vi "ESP32 Continuous Serial Write and Read - Modified.vi"() -> ()   [LabVIEW 2022 SP3]
doc: "This example performs writes and reads on a serial port, as directed by the user. You can press the Write and Read buttons, and change the Read Count, while the example is running.\n\nThe parameters set for the serial port must match the parameters of the connected instrument or device. In this example, the Read Count parameter specifies the number of bytes that the serial port reads. If there were more bytes at the port than the specified number, those bytes would not be read. If there were less bytes at the port than the specified number, you would receive a timeout error.\n\nThis example expands upon the flow control options for XON and XOFF, allowing the user to choose those control characters. Also, the user can enable or disable a termination character. Some devices require a termination character in order to identify the end of command strings. Some devices send a termination character to signify the end of data to be read. This example shows how you can end the Read operation once a termination character is detected in the buffer and/or append a termination character at the end of the Write data."
uses:
  Serial - Settings.ctl
  Serial - XON-XOFF Characters.ctl
  Serial - ASCII Characters.ctl
  ESP32-PSOC-State Machine.ctl
  <vilib>/Instr/_visa.llb/VISA Flush IO Buffer Mask.ctl
  <vilib>/Instr/_visa.llb/VISA Configure Serial Port (Instr).vi
panel:
  in  "Difficulty":T1
  out "error":bool
  out "Connected":bool
  out "Serial Settings:Number of Bytes at Serial Port":u32
  out "Response 2":string
  in  "Toggle LED":bool
  in  "Enum":T2
  in  "Termination Character":u8=10 format="%.0x"
  in  "End Write on Termination Character?":bool=TRUE
  in  "Stop":bool
  out "Read Count":u32=1000
  out "Response":string
  in  "XON/XOFF Characters":T3={"XON"=enum."DC1", "XOFF"=enum."DC3"}
  in  "Serial Settings":T5={"baud rate"=115200, "data bits"=8, "parity"=enum."None", "stop bits"=10, "flow control"=0} {"flow control" items=["None"=0, "XON/XOFF"=1, "RTS/CTS"=2, "DTR/DSR"=4]; "stop bits" items=["1.0"=10, "1.5"=15, "2.0"=20]; "data bits" min=5 max=8 step=1; "baud rate" items=["75"=75, "110"=110, "134"=134, "150"=150, "300"=300, "600"=600, "1200"=1200, "1800"=1800, "2400"=2400, "4800"=4800, "7200"=7200, "9600"=9600, "14400"=14400, "19200"=19200, "28800"=28800, "38400"=38400, "56000"=56000, "57600"=57600, "115200"=115200, "128000"=128000, "230400"=230400]}
  in  "End Read on Termination Character?":bool=TRUE
  in  "VISA resource name":refnum<visa-resource-name>="COM4"
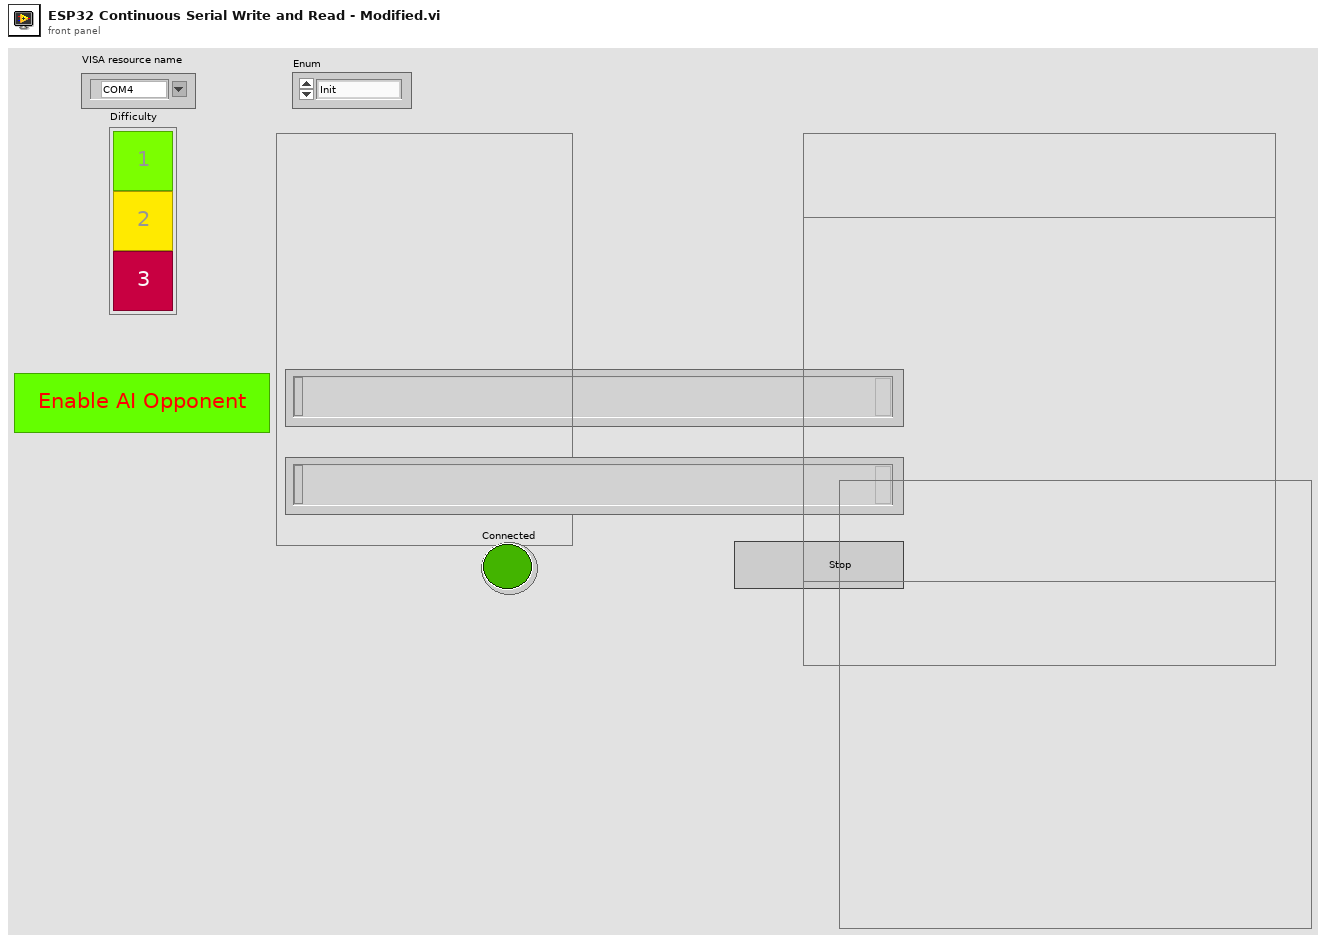
[diagram p1: front panel]
types:
  T1 = cluster{"Command A":bool, "Command B":bool, "Command C":bool}
  T2 = typedef "ESP32-PSOC-State Machine.ctl" = enum8{"Init", "Connect", "idle", "send", "wait", "receive", "que", "error", "exit"}
  T3 = typedef "Serial - XON-XOFF Characters.ctl" = cluster{"XON":T4, "XOFF":T4}
  T4 = typedef "Serial - ASCII Characters.ctl" = enum16{"NUL", "SOH", "STX", "ETX", "EOT", "ENQ", "ACK", "BEL", "BS", "HT", "LF", "VT", "FF", "CR", "SO", "SI", "DLE", "DC1", "DC2", "DC3", "DC4", "NAK", "SYN", "ETB", "CAN", "EM", "SUB", "ESC", "FS", "GS", "RS", "US", "SP", "!", "\"", "#", "$", "%", "&", "'", "(", ")", "*", "+", ",", "- (-)", ".", "/", "0", "1", "2", "3", "4", "5", "6", "7", "8", "9", ":", ";", "<", "=", ">", "?", "@", "A", "B", "C", "D", "E", "F", "G", "H", "I", "J", "K", "L", "M", "N", "O", "P", "Q", "R", "S", "T", "U", "V", "W", "X", "Y", "Z", "[", "\\", "]", "^", "_", "`", "a", "b", "c", "d", "e", "f", "g", "h", "i", "j", "k", "l", "m", "n", "o", "p", "q", "r", "s", "t", "u", "v", "w", "x", "y", "z", "{", "|", "}", "~"}
  T5 = typedef "Serial - Settings.ctl" = cluster{"baud rate":u32, "data bits":u16, "parity":enum16{"None", "Odd", "Even", "Mark", "Space"}, "stop bits":u16, "flow control":u16}
  T6 = typedef "VISA Flush IO Buffer Mask.ctl" = u16
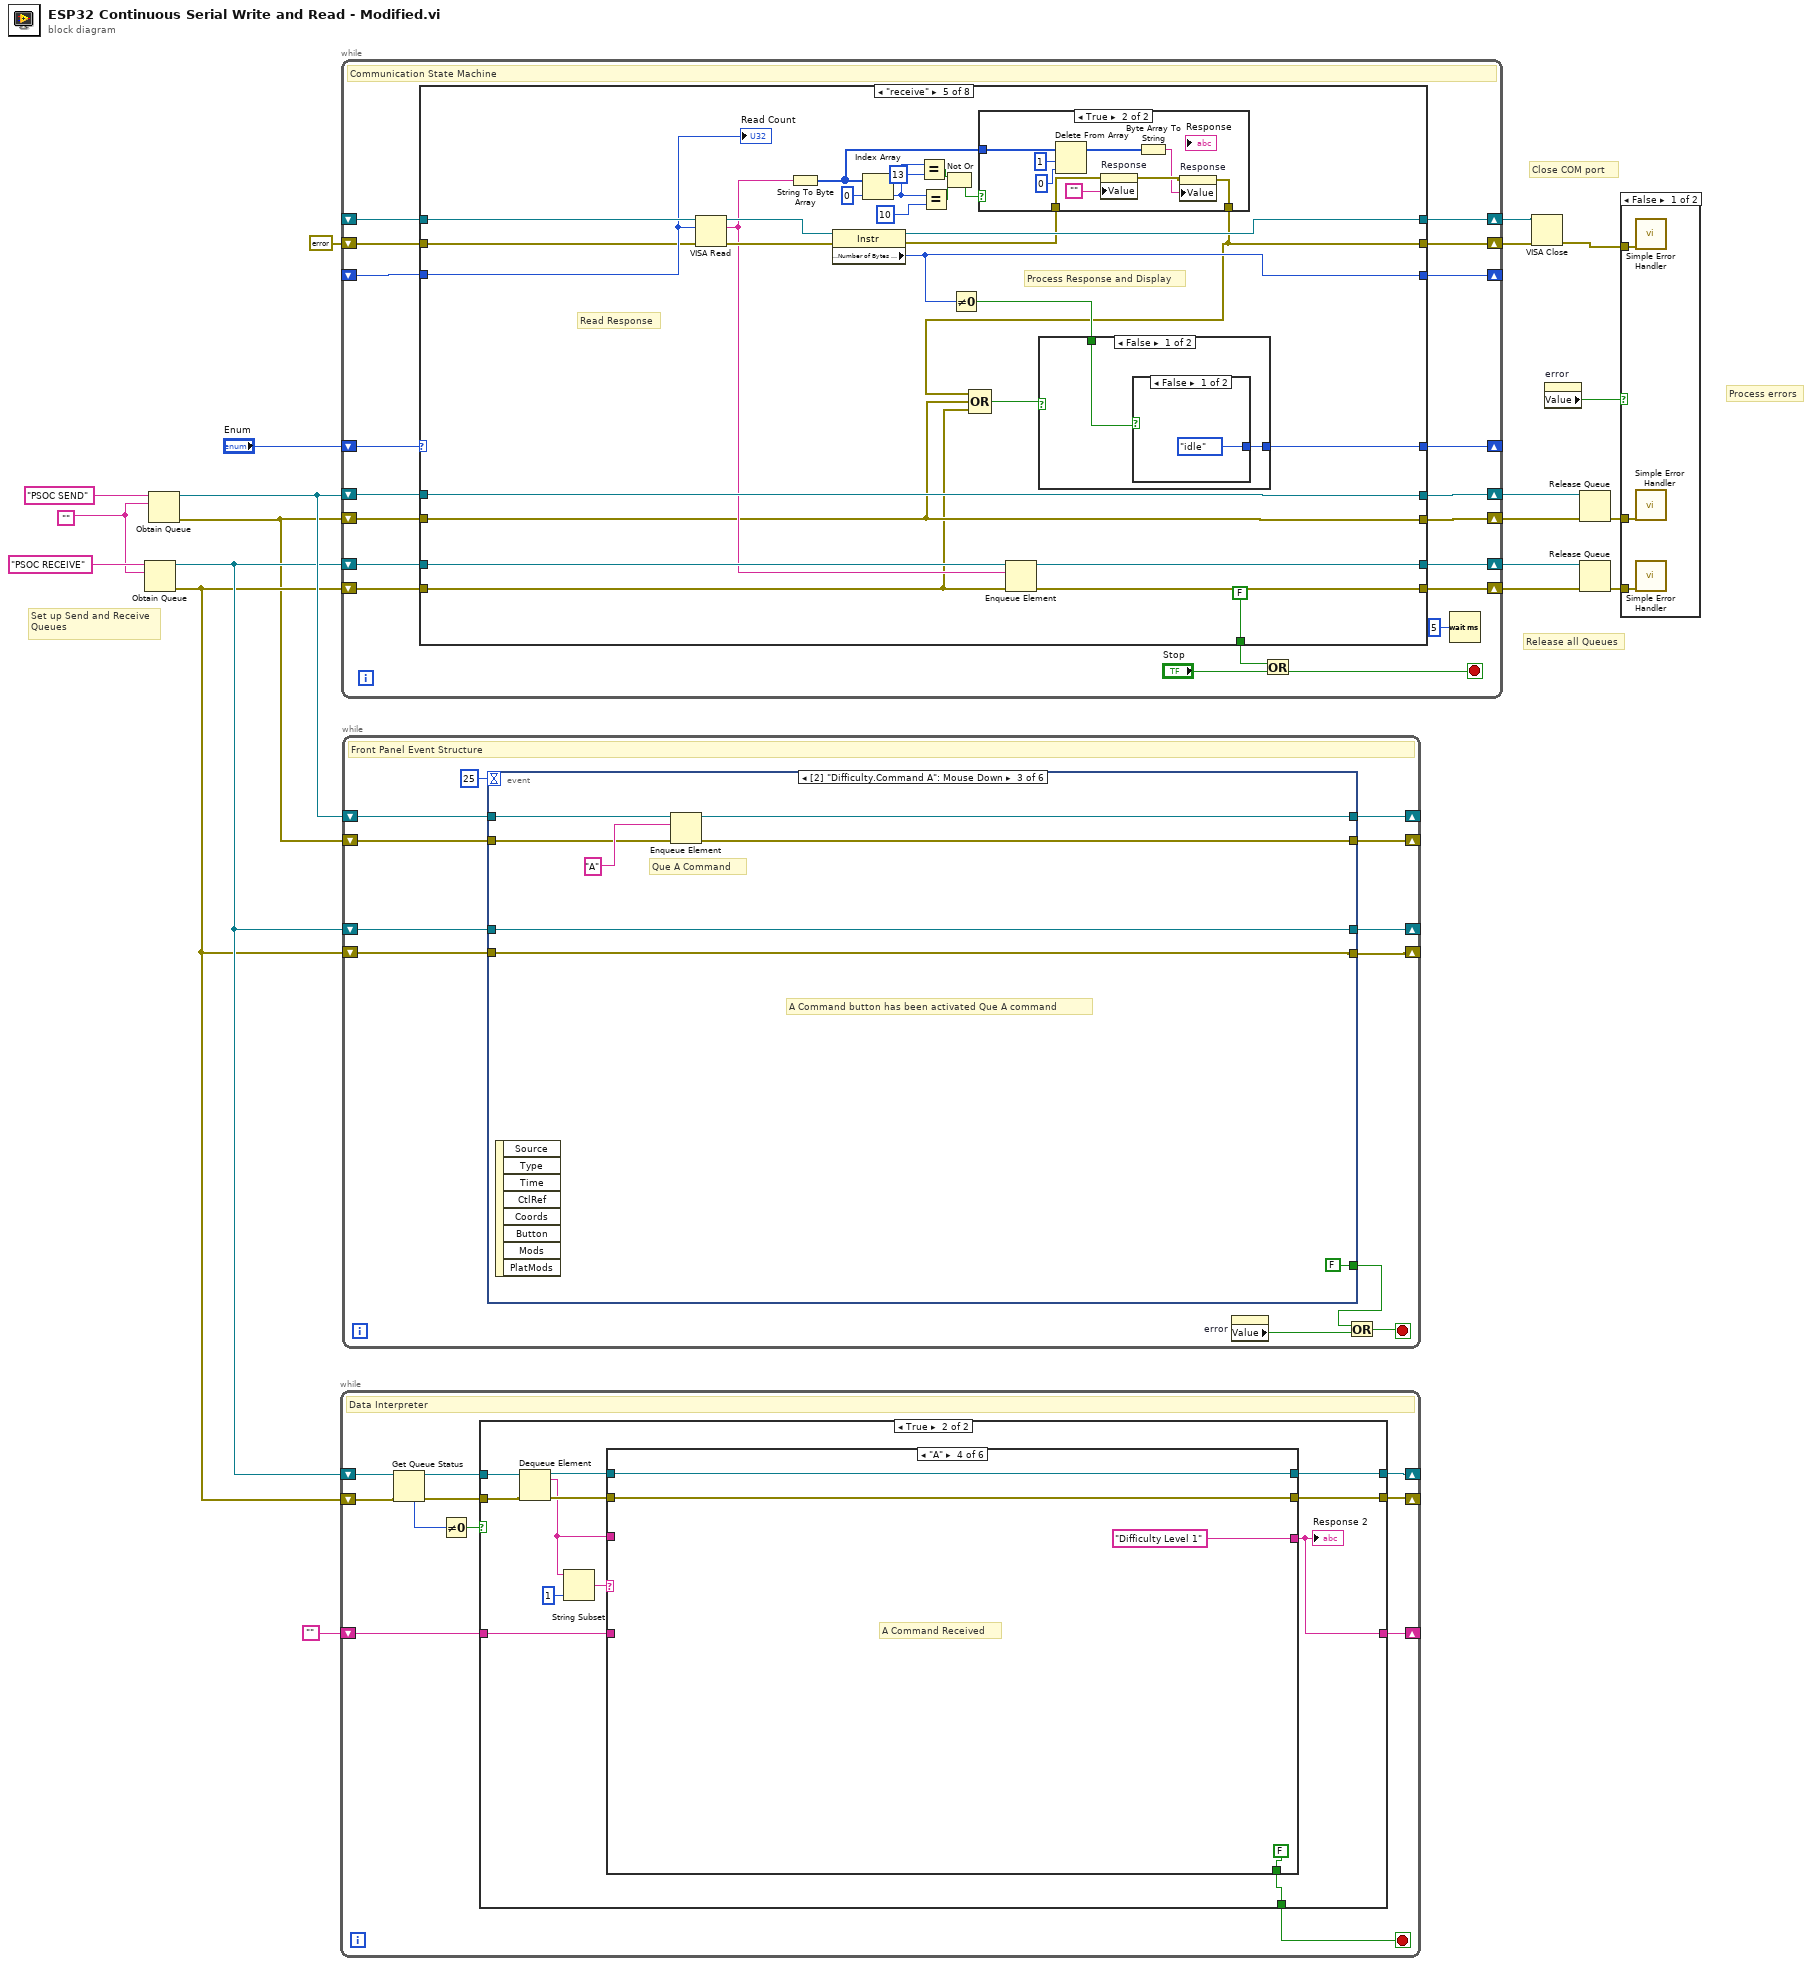
[diagram p0: block diagram]
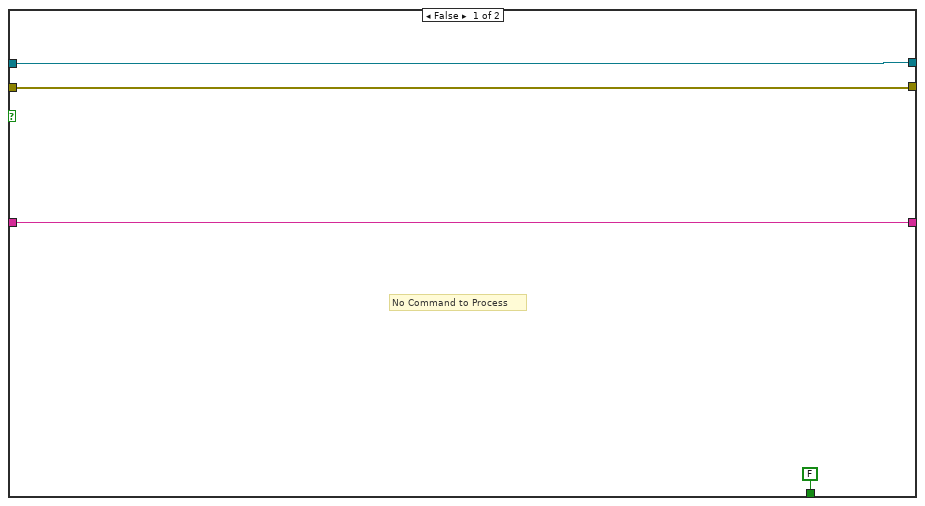
[diagram p3: hidden frame]
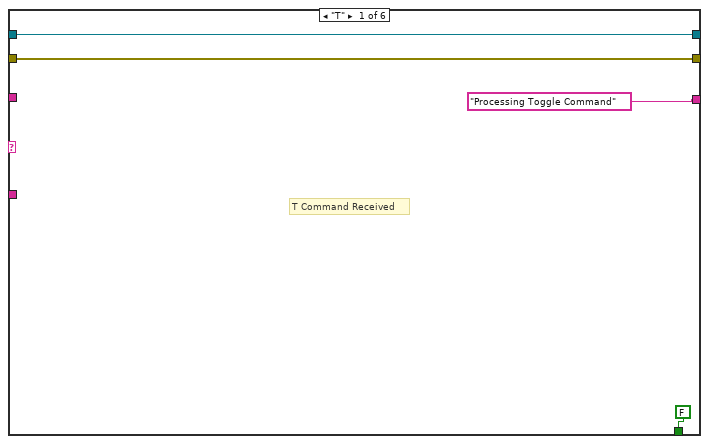
[diagram p4: hidden frame]
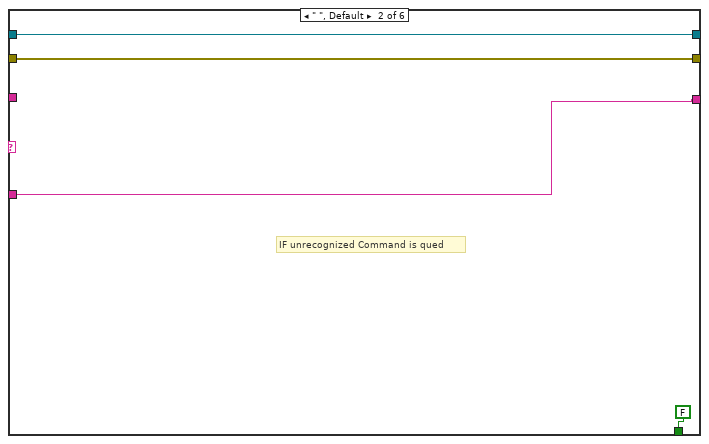
[diagram p5: hidden frame]
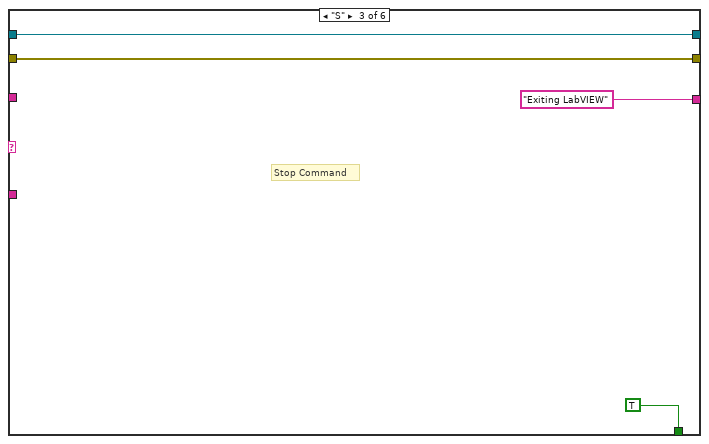
[diagram p6: hidden frame]
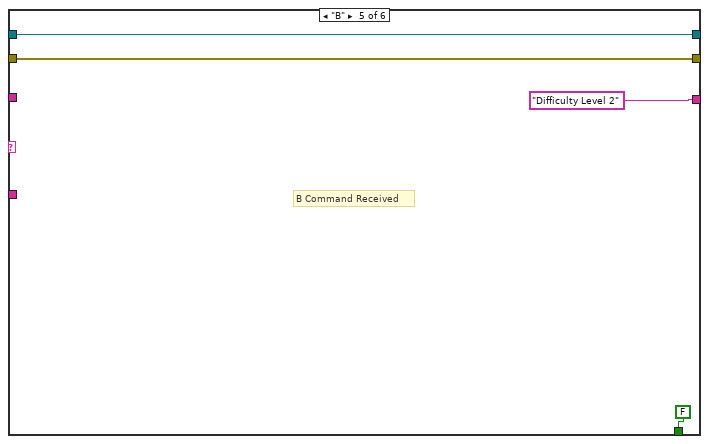
[diagram p7: hidden frame]
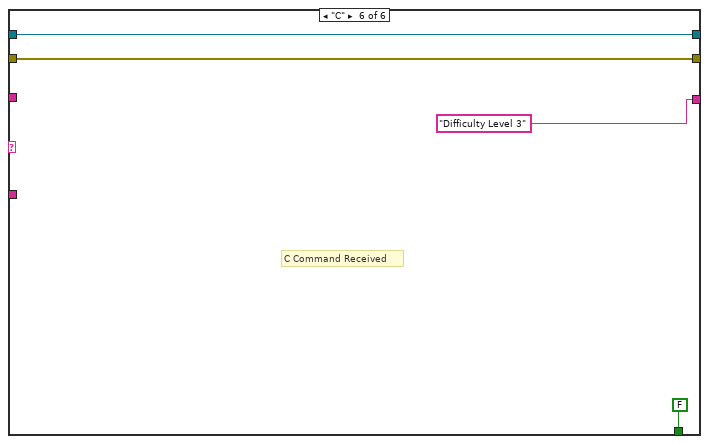
[diagram p8: hidden frame]
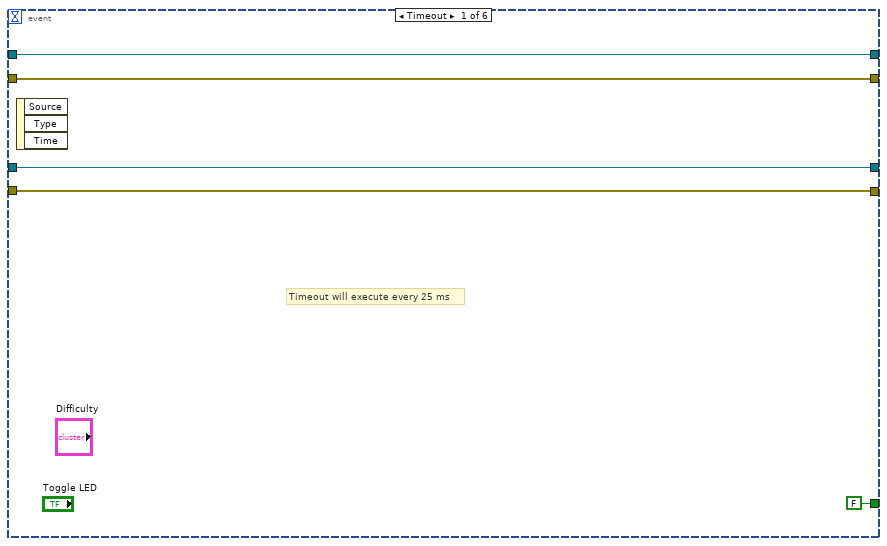
[diagram p9: hidden frame]
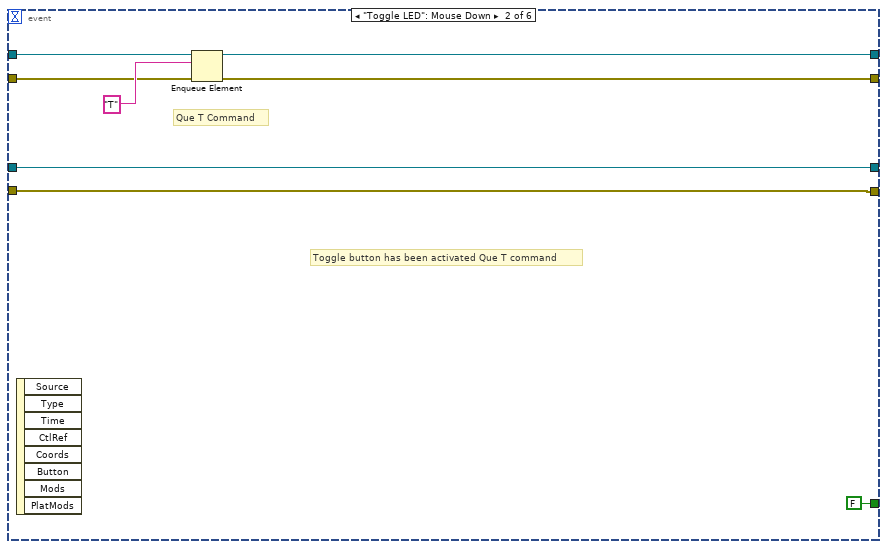
[diagram p10: hidden frame]
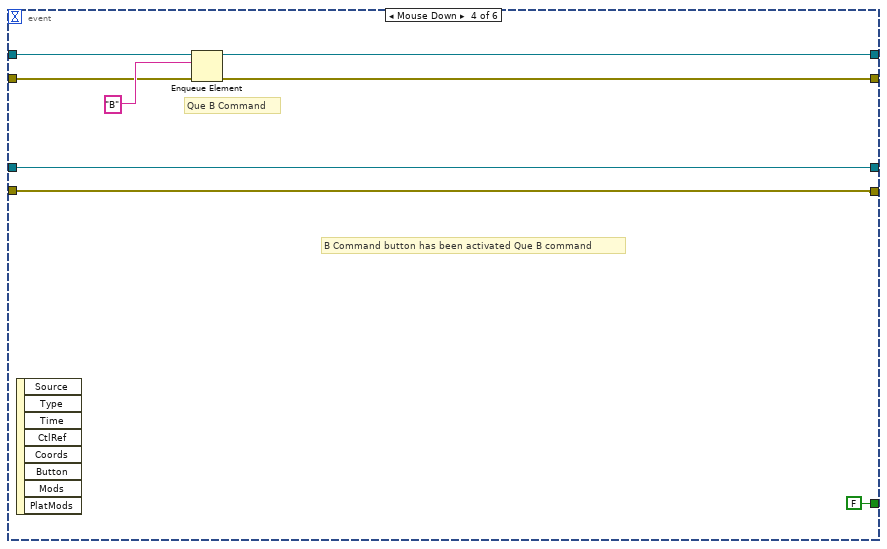
[diagram p11: hidden frame]
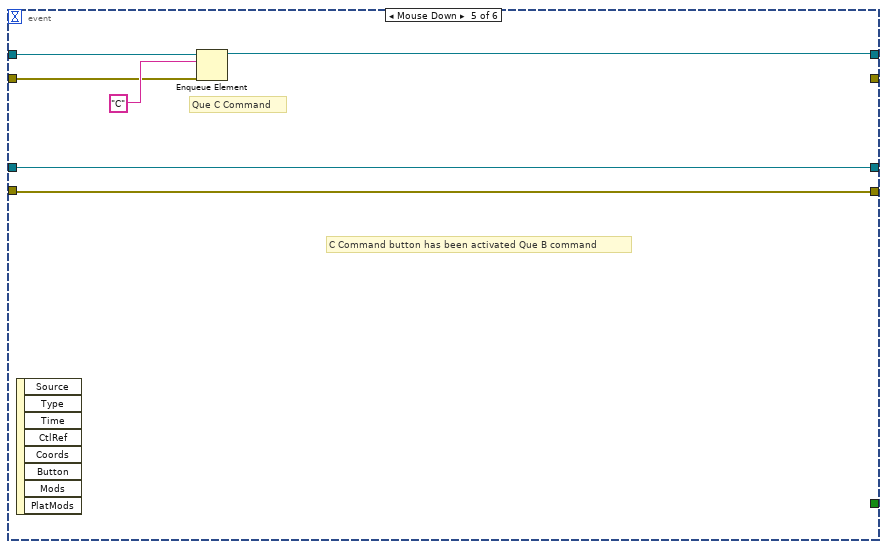
[diagram p12: hidden frame]
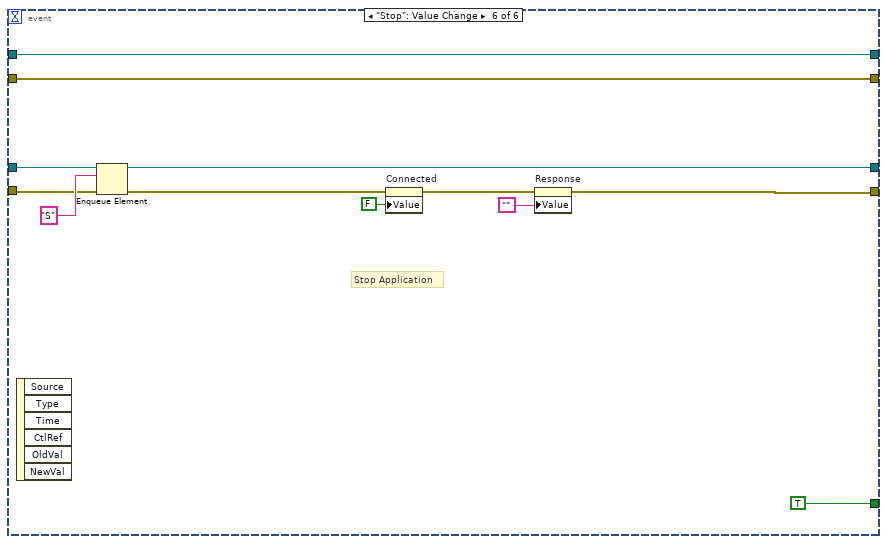
[diagram p13: hidden frame]
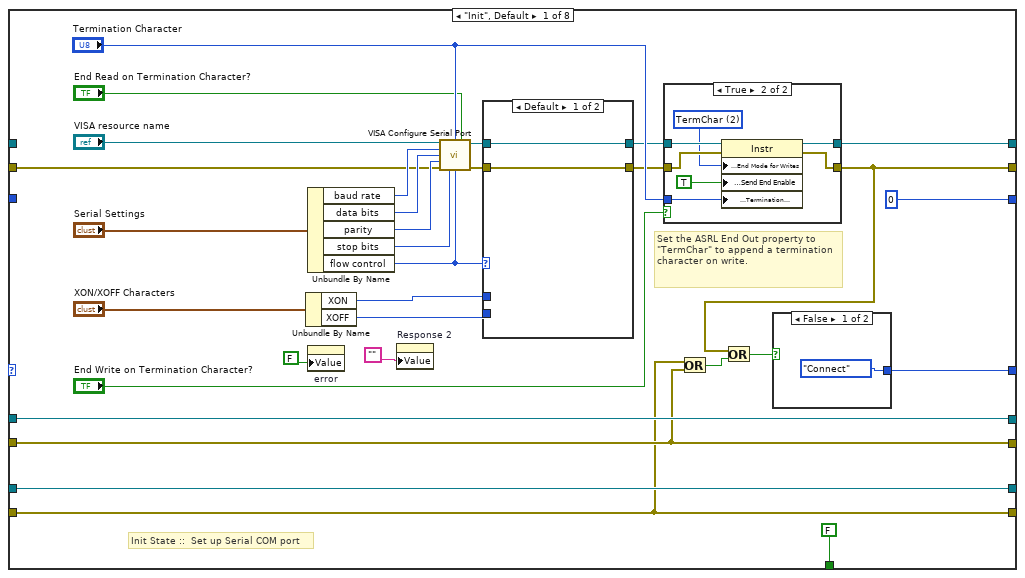
[diagram p14: hidden frame]
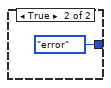
[diagram p15: hidden frame]
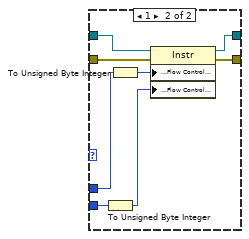
[diagram p17: hidden frame]
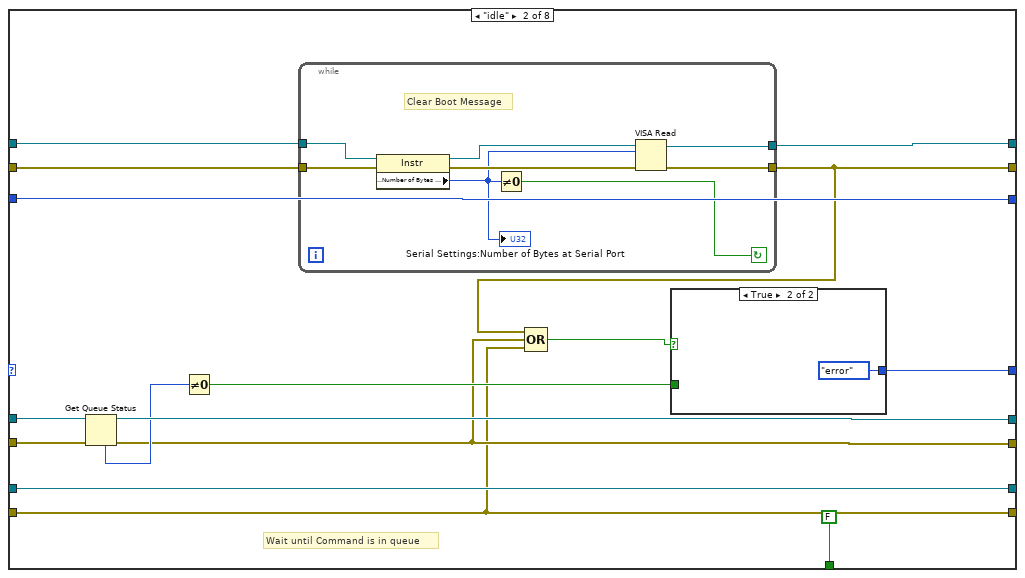
[diagram p18: hidden frame]
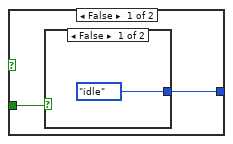
[diagram p19: hidden frame]
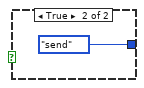
[diagram p20: hidden frame]
diagram:
  w10 = ""
  # "Process errors"
  # "Release all Queues"
  # "Close COM port"
  # "Set up Send and Receive\nQueues"
  n1 = Obtain Queue(name (unnamed)="PSOC RECEIVE", element data type=w10) -> (queue out=w9:refnum<queue>, error out=w8:errorcluster)  [unwired: 3 in, 1 out]
  n2 = Obtain Queue(name (unnamed)="PSOC SEND", element data type=w10) -> (queue out=w12:refnum<queue>, error out=w2:errorcluster)  [unwired: 3 in, 1 out]
  n3 = while {
    shift-right: [w25] -> _
    shift-left: w9 -> [w31]
    shift-right: [w24] -> _
    shift-left: w8 -> [w30]
    shift-right: [w22] -> _
    shift-left: "" -> [w21]
    stop <- w23 stop-if-true
    # "Data Interpreter"
    n4 = Get Queue Status(queue=w31, error in (no error)=w30) -> (queue out=w27:refnum<queue>, error out=w26:errorcluster, # elements in queue=w29:i32)  [unwired: 1 in, 5 out]
    n5 = Not Equal To 0?(x=w29) -> (x != 0?=w28:bool)
    n6 = case shown="True" w28 {
      tunnel: w27 -> [w35 w47]
      tunnel: w26 -> [w34 w46]
      tunnel: [w35 w41] -> w25
      tunnel: [w34 w40] -> w24
      tunnel: [FALSE w39] -> w23
      tunnel: [w32 w37] -> w22
      tunnel: w21 -> [w32 w36]
      frame False {
        # "No Command to Process"
      }
      frame True {
        n7 = Dequeue Element(queue=w47, error in (no error)=w46) -> (queue out=w45:refnum<queue>, element=w38:string, error out=w44:errorcluster)  [unwired: 1 in, 1 out]
        n8 = String Subset(string=w38, length (rest)=1 ("length (rest)")) -> (substring=w42:string)  [unwired: 1 in]
        n9 = case shown="\"A\"" w42 {
          tunnel: w45 -> [w51 w55 w59 w63 w67 w69]
          tunnel: w44 -> [w50 w54 w58 w62 w66 w70]
          tunnel: [w51 w55 w59 w63 w67 w69] -> w41
          tunnel: [w50 w54 w58 w62 w66 w70] -> w40
          tunnel: w38 -> [_ _ _ _ _ _]
          tunnel: [FALSE FALSE TRUE FALSE FALSE FALSE] -> w39
          tunnel: ["Processing Toggle Command" w52 "Exiting LabVIEW" "Difficulty Level 1" "Difficulty Level 2" "Difficulty Level 3"] -> w37
          tunnel: w36 -> [_ w52 _ _ _ _]
          frame "T" {
            # "T Command Received"
          }
          frame " ", Default {
            # "IF unrecognized Command is qued"
          }
          frame "S" {
            # "Stop Command"
          }
          frame "A" {
            # "A Command Received"
          }
          frame "B" {
            # "B Command Received"
          }
          frame "C" {
            # "C Command Received"
          }
        }
        "Response 2" <- w37
      }
    }
  }
  n10 = while {
    shift-right: [w83] -> w20
    shift-left: w12 -> [w91]
    shift-right: [w82] -> w18
    shift-left: w2 -> [w90]
    shift-right: [w81] -> w19
    shift-left: w9 -> [w89]
    shift-right: [w80] -> w15
    shift-left: w8 -> [w88]
    shift-right: [w75] -> _
    shift-left: "Enum" -> [w74]
    shift-right: [w87] -> w14
    shift-left: _ -> [w84]
    shift-right: [w86] -> w13
    shift-left: errorcluster {"status"=FALSE, "code"=0, "source"=""} ("error out") -> [w85]
    shift-right: [w79] -> _
    shift-left: _ -> [w78]
    stop <- w73 stop-if-true
    # "Communication State Machine"
    n11 = case shown="\"receive\"" w74 {
      selector: w74 -> [_ _ _ _ _ _ w291 _]
      tunnel: [w121 w157 w196 w213 w250 w275 w290 w313] -> w83
      tunnel: [w95 w147 w187 w207 w232 w272 w289 w312] -> w82
      tunnel: [w101 w155 w188 w216 w251 ESP32-PSOC-State_Machine."exit" ("Enum") w291 ESP32-PSOC-State_Machine."idle" ("Enum")] -> w75
      tunnel: w91 -> [w121 w159 w198 w213 w250 w275 w290 w313]
      tunnel: w90 -> [w95 w158 w197 w207 w232 w272 w289 w312]
      tunnel: w89 -> [w122 w153 w195 w210 w245 w274 w288 w311]
      tunnel: w88 -> [w94 w146 w186 w206 w231 w271 w279 w310]
      tunnel: [w103 w150 w182 w215 w240 w277 w294 w315] -> w87
      tunnel: [w97 w148 w183 w208 w233 w273 w293 w316] -> w86
      tunnel: w85 -> [w99 w149 w191 w214 w235 w273 w293 w317]
      tunnel: w84 -> [_ w151 w193 w204 w248 w277 w294 w318]
      tunnel: [w122 w153 w195 w210 w243 w274 w286 w311] -> w81
      tunnel: [w94 w146 w186 w206 w244 w271 w282 w310] -> w80
      tunnel: [u32 0 ("Bytes at Port") w152 w194 w212 w246 w276 w292 w314] -> w79
      tunnel: w78 -> [_ w152 w194 _ w242 w276 w292 w314]
      tunnel: [FALSE FALSE FALSE FALSE FALSE FALSE TRUE FALSE] -> w72
      frame "Init", Default {
        # "Init State ::  Set up Serial COM port"
        # "Set the ASRL End Out property to \"TermChar\" to append a termination character on write."
        n12 = Unbundle By Name("XON/XOFF Characters") -> ("XON"=w115:T4, "XOFF"=w116:T4)
        n13 = Unbundle By Name("Serial Settings") -> ("baud rate"=w111:u32, "data bits"=w110:u16, "parity"=w109:enum16{"None", "Odd", "Even", "Mark", "Space"}, "stop bits"=w108:u16, "flow control"=w114:u16)
        n14 = property on="error" class="Bool (strict)"("Value"=FALSE ("error")) -> ()  [unwired: 2 in, 2 out]
        n15 = property on="Response 2" class="Str"("Value"="") -> ()  [unwired: 2 in, 2 out]
        n16 = call-poly "VISA Configure Serial Port"("VISA resource name"="VISA resource name", "termination char\n(0xA = '\\n' = LF)"="Termination Character", "Enable Termination\nChar (T)"="End Read on Termination Character?", "baud rate (9600)"=w111, "data bits (8)"=w110, "parity (0:none)"=w109, "error in (no error)"=w99, "stop bits (10: 1 bit)"=w108, "flow control (0:none)"=w114) -> ("VISA resource name out"=w107:refnum<visa-resource-name>, "error out"=w106:errorcluster)  [unwired: 1 in, 4 out]
        n17 = case shown="Default" w114 {
          tunnel: [w134 w143] -> w117
          tunnel: [w135 w142] -> w118
          tunnel: w106 -> [w134 w141]
          tunnel: w107 -> [w135 w140]
          tunnel: w115 -> [_ w139]
          tunnel: w116 -> [_ w138]
          frame Default {
          }
          frame 1 {
            n18 = To Unsigned Byte Integer(number=w138) -> (unsigned 8bit integer=w137:u8)
            n19 = To Unsigned Byte Integer(number=w139) -> (unsigned 8bit integer=w136:u8)
            n20 = property class="Instr"(reference=w140, error in=w141, "Serial Settings:Flow Control XON Character"=w136, "Serial Settings:Flow Control XOFF Character"=w137) -> (reference out=w142:refnum<visa-resource-name>, error out=w143:errorcluster)
          }
        }
        n21 = case shown="True" "End Write on Termination Character?" {
          tunnel: w118 -> [w125 w133]
          tunnel: w117 -> [w126 w132]
          tunnel: [w125 w131] -> w103
          tunnel: [w126 w130] -> w97
          tunnel: "Termination Character" -> [_ w128]
          frame False {
          }
          frame True {
            w129 = u16 2 items=["None", "LastBit", "TermChar", "Break"] ("Serial Settings:Serial End Mode for Writes")
            n22 = property class="Instr"(reference=w133, error in=w132, "Serial Settings:End Mode for Writes"=w129, "Message Based Settings:Send End Enable"=TRUE, "Message Based Settings:Termination Character"=w128) -> (reference out=w131:refnum<visa-resource-name>, error out=w130:errorcluster)
          }
        }
        n23 = Or(x=w94, y=w95) -> (x .or. y?=w96:bool)
        n24 = Or(x=w97, y=w96) -> (x .or. y?=w98:bool)
        n25 = case shown="False" w98 {
          tunnel: [ESP32-PSOC-State_Machine."Connect" ("Enum") ESP32-PSOC-State_Machine."error" ("Enum")] -> w101
          frame False {
          }
          frame True {
          }
        }
      }
      frame "idle" {
        # "Wait until Command is in queue"
        n26 = Get Queue Status(queue=w159, error in (no error)=w158) -> (queue out=w157:refnum<queue>, error out=w147:errorcluster, # elements in queue=w156:i32)  [unwired: 1 in, 5 out]
        n27 = Not Equal To 0?(x=w156) -> (x != 0?=w154:bool)
        n28 = while {
          tunnel: w151 -> [w172]
          tunnel: [w168] -> w150
          tunnel: w149 -> [w171]
          tunnel: [w166] -> w148
          stop <- w170 continue-if-true
          # "Clear Boot Message"
          n29 = property class="Instr"(reference=w172, error in=w171) -> (reference out=w169:refnum<visa-resource-name>, error out=w167:errorcluster, "Serial Settings:Number of Bytes at Serial Port"=w165:u32)
          "Serial Settings:Number of Bytes at Serial Port" <- w165
          n30 = Not Equal To 0?(x=w165) -> (x != 0?=w170:bool)
          n31 = VISA Read(VISA resource name=w169, byte count=w165, error in (no error)=w167) -> (VISA resource name out=w168:refnum<visa-resource-name>, error out=w166:errorcluster)  [unwired: 2 out]
        }
        n32 = Compound Arithmetic op=OR(w148, w147, w146) -> (w145:bool)
        n33 = case shown="True" w145 {
          tunnel: [w161 ESP32-PSOC-State_Machine."error" ("Enum")] -> w155
          tunnel: w154 -> [w160 _]
          frame False {
            n34 = case shown="False" w160 {
              tunnel: [ESP32-PSOC-State_Machine."idle" ("Enum") ESP32-PSOC-State_Machine."send" ("Enum")] -> w161
              frame False {
              }
              frame True {
              }
            }
          }
          frame True {
          }
        }
      }
      frame "send" {
        w189 = T6 64 items=["Flush Receive Buffer"=16, "Write Transmit Buffer to Device"=32, "Flush Receive Buffer (No I/O)"=64, "Flush Transmit Buffer"=128] ("Mask")
        # "Read and Discard Echo Command"
        # "Wait for Response"
        # "Send Command"
        n35 = Dequeue Element(queue=w198, error in (no error)=w197) -> (queue out=w196:refnum<queue>, element=w176:string, error out=w187:errorcluster)  [unwired: 1 in, 1 out]
        n36 = VISA Flush I/O Buffer(VISA resource name=w193, mask (16)=w189, error in (no error)=w191) -> (VISA resource name out=w192:refnum<visa-resource-name>, error out=w190:errorcluster)
        n37 = Concatenate Strings(w176, "\r\n") -> (w175:string)
        n38 = VISA Write(VISA resource name=w192, write buffer=w175, error in (no error)=w190) -> (VISA resource name out=w174:refnum<visa-resource-name>, error out=w180:errorcluster)  [unwired: 1 out]
        n39 = flat-sequence {
          tunnel: w174 -> [w200]
          tunnel: [w200] -> w173
          frame #0 {
            n40 = Wait (ms)(milliseconds to wait=u32 15) -> ()  [unwired: 1 out]
          }
        }
        n41 = property class="Instr"(reference=w173, error in=w180) -> (reference out=w181:refnum<visa-resource-name>, error out=w179:errorcluster, "Serial Settings:Number of Bytes at Serial Port"=w178:u32)
        n42 = VISA Read(VISA resource name=w181, byte count=w178, error in (no error)=w179) -> (VISA resource name out=w182:refnum<visa-resource-name>, error out=w183:errorcluster)  [unwired: 2 out]
        n43 = Compound Arithmetic op=OR(w183, w187, w186) -> (w185:bool)
        n44 = case shown="False" w185 {
          tunnel: [ESP32-PSOC-State_Machine."wait" ("Enum") ESP32-PSOC-State_Machine."error" ("Enum")] -> w188
          frame False {
          }
          frame True {
          }
        }
      }
      frame "wait" {
        # "Wait for actual Response"
        n45 = flat-sequence {
          tunnel: w204 -> [w218]
          tunnel: [w218] -> w203
          frame #0 {
            n46 = Wait (ms)(milliseconds to wait=u32 15) -> ()  [unwired: 1 out]
          }
        }
        n47 = property class="Instr"(reference=w203, error in=w214) -> (reference out=w215:refnum<visa-resource-name>, error out=w208:errorcluster, "Serial Settings:Number of Bytes at Serial Port"=w212:u32)
        n48 = Not Equal To 0?(x=w212) -> (x != 0?=w211:bool)
        n49 = Compound Arithmetic op=OR(w208, w207, w206) -> (w209:bool)
        n50 = case shown="False" w209 {
          tunnel: [w220 ESP32-PSOC-State_Machine."error" ("Enum")] -> w216
          tunnel: w211 -> [w219 _]
          frame False {
            n51 = case shown="True" w219 {
              tunnel: [ESP32-PSOC-State_Machine."wait" ("Enum") ESP32-PSOC-State_Machine."receive" ("Enum")] -> w220
              frame False {
              }
              frame True {
              }
            }
          }
          frame True {
          }
        }
      }
      frame "receive" {
        # "Process Response and Display"
        # "Read Response"
        n52 = VISA Read(VISA resource name=w248, byte count=w242, error in (no error)=w235) -> (VISA resource name out=w241:refnum<visa-resource-name>, read buffer=w237:string, error out=w247:errorcluster)  [unwired: 1 out]
        n53 = String To Byte Array(string=w237) -> (unsigned byte array=w236:u8[])
        n54 = property class="Instr"(reference=w241, error in=w247) -> (reference out=w240:refnum<visa-resource-name>, error out=w234:errorcluster, "Serial Settings:Number of Bytes at Serial Port"=w246:u32)
        n55 = Index Array(array=w236, index=0) -> (element=w228:u8)
        n56 = Equal?(x=w228, y=u8 13) -> (x = y?=w226:bool)
        n57 = Equal?(x=w228, y=u8 10) -> (x = y?=w225:bool)
        n58 = Not Or(1:w225, 2:w226) -> (0:w224:bool)
        n59 = Not Equal To 0?(x=w246) -> (x != 0?=w249:bool)
        n60 = case shown="True" w224 {
          tunnel: w236 -> [_ w266]
          tunnel: w234 -> [w257 w259]
          tunnel: [w257 w258] -> w233
          frame False {
          }
          frame True {
            n61 = Delete From Array(array=w266, length=1, index=0) -> (array with subset deleted=w263:u8[])  [unwired: 1 out]
            n62 = property on="Response" class="Str"(error in=w259, "Value"="") -> (error out=w261:errorcluster)  [unwired: 1 in, 1 out]
            n63 = Byte Array To String(unsigned byte array=w263) -> (string=w260:string)
            n64 = property on="Response" class="Str"(error in=w261, "Value"=w260) -> (error out=w258:errorcluster)  [unwired: 1 in, 1 out]
          }
        }
        n65 = Compound Arithmetic op=OR(w233, w232, w231) -> (w230:bool)
        n66 = Enqueue Element(queue=w245, element=w237, error in (no error)=w231) -> (queue out=w243:refnum<queue>, error out=w244:errorcluster)  [unwired: 1 in, 1 out]
        n67 = case shown="False" w230 {
          tunnel: [w253 ESP32-PSOC-State_Machine."error" ("Enum")] -> w251
          tunnel: w249 -> [w252 _]
          frame False {
            n68 = case shown="False" w252 {
              tunnel: [ESP32-PSOC-State_Machine."idle" ("Enum") ESP32-PSOC-State_Machine."receive" ("Enum")] -> w253
              frame False {
              }
              frame True {
              }
            }
          }
          frame True {
          }
        }
        "Read Count" <- w242
      }
      frame "error" {
        # "Process any error"
        n69 = Build Array(w273, w272, w271) -> (w270:errorcluster[])
        n70 = for {
          tunnel: w270 -> [w278] mode=indexing
          n71 = call <vilib>:"General Error Handler.vi"("error in (no error)"=w278) -> ()  [unwired: 10 in, 5 out]
        }
        "error" <- TRUE ("error")
      }
      frame "exit" {
        # "Exit due to error"
        n72 = Enqueue Element(queue=w288, element="S", error in (no error)=w279) -> (queue out=w286:refnum<queue>, error out=w284:errorcluster)  [unwired: 1 in, 1 out]
        n73 = property on="Connected" class="Bool (strict)"(error in=w284, "Value"=FALSE ("Connected")) -> (error out=w283:errorcluster)  [unwired: 1 in, 1 out]
        n74 = property on="Response" class="Str"(error in=w283, "Value"="") -> (error out=w282:errorcluster)  [unwired: 1 in, 1 out]
      }
      frame "Connect" {
        # "Validating connection"
        # "Send ID to validate connection"
        # "Clear any residual characters"
        n75 = while {
          shift-right: [w342] -> w306
          shift-left: w317 -> [w348]
          shift-right: [w341] -> w307
          shift-left: w318 -> [w347]
          stop <- w346 continue-if-true
          n76 = property class="Instr"(reference=w347, error in=w348) -> (reference out=w344:refnum<visa-resource-name>, error out=w343:errorcluster, "Bytes at Port"=w340:u32)
          n77 = VISA Read(VISA resource name=w344, byte count=w340, error in (no error)=w343) -> (VISA resource name out=w341:refnum<visa-resource-name>, read buffer=w339:string, error out=w342:errorcluster)  [unwired: 1 out]
          n78 = Wait (ms)(milliseconds to wait=u32 5) -> ()  [unwired: 1 out]
          n79 = Search/Split String(string=w339, search string/char (-)="Commands") -> (match + rest of string=w337:string)  [unwired: 1 in, 2 out]
          n80 = String Length(string=w337) -> (length=w336:i32)
          n81 = Equal To 0?(x=w336) -> (x = 0?=w346:bool)
        }
        n82 = Concatenate Strings("I" ("write buffer"), "\r\n") -> (w295:string)
        n83 = VISA Write(VISA resource name=w307, write buffer=w295, error in (no error)=w306) -> (VISA resource name out=w301:refnum<visa-resource-name>, error out=w305:errorcluster)  [unwired: 1 out]
        n84 = flat-sequence {
          tunnel: w301 -> [w335]
          tunnel: [w335] -> w300
          frame #0 {
            n85 = Wait (ms)(milliseconds to wait=u32 5) -> ()  [unwired: 1 out]
          }
        }
        n86 = property class="Instr"(reference=w300, error in=w305) -> (reference out=w303:refnum<visa-resource-name>, error out=w304:errorcluster, "Bytes at Port"=w302:u32)
        n87 = VISA Read(VISA resource name=w303, byte count=w302, error in (no error)=w304) -> (VISA resource name out=w298:refnum<visa-resource-name>, error out=w299:errorcluster)  [unwired: 2 out]
        n88 = while {
          shift-right: [w322] -> w316
          shift-left: w299 -> [w328]
          shift-right: [w323] -> w315
          shift-left: w298 -> [w321]
          stop <- w319 stop-if-true
          n89 = flat-sequence {
            tunnel: w321 -> [w333]
            tunnel: [w333] -> w320
            frame #0 {
              n90 = Wait (ms)(milliseconds to wait=u32 15) -> ()  [unwired: 1 out]
            }
          }
          n91 = property class="Instr"(reference=w320, error in=w328) -> (reference out=w326:refnum<visa-resource-name>, error out=w327:errorcluster, "Bytes at Port"=w325:u32)
          n92 = VISA Read(VISA resource name=w326, byte count=w325, error in (no error)=w327) -> (VISA resource name out=w323:refnum<visa-resource-name>, read buffer=w324:string, error out=w322:errorcluster)  [unwired: 1 out]
          n93 = Search/Split String(string=w324, search string/char (-)="IESP32") -> (match + rest of string=w330:string)  [unwired: 1 in, 2 out]
          n94 = String Length(string=w330) -> (length=w329:i32)
          n95 = Not Equal To 0?(x=w329) -> (x != 0?=w319:bool)
          "Connected" <- w319
        }
      }
    }
    n96 = Or(x=w72, y="Stop") -> (x .or. y?=w73:bool)
    n97 = Wait (ms)(milliseconds to wait=u32 5) -> ()  [unwired: 1 out]
  }
  n98 = while {
    shift-right: [w357] -> _
    shift-left: w12 -> [w358]
    shift-right: [w356] -> _
    shift-left: w2 -> [w359]
    shift-right: [w349] -> _
    shift-left: w9 -> [w355]
    shift-right: [w353] -> _
    shift-left: w8 -> [w354]
    stop <- w350 stop-if-true
    # "Front Panel Event Structure"
    n99 = event shown="[2] \"Difficulty.Command A\": Mouse Down" {
      selector: _ -> [_ _ _ _ _ _]
      dyn-events: _ -> [_ _ _ _ _ _]
      timeout: 25 -> [_ _ _ _ _ _]
      tunnel: w359 -> [w363 w371 w379 w387 w390 w405]
      tunnel: w358 -> [w364 w373 w381 w389 w391 w406]
      tunnel: [w364 w370 w378 w386 w392 w406] -> w357
      tunnel: [w363 w369 w377 w385 _ w405] -> w356
      tunnel: [FALSE FALSE FALSE FALSE _ TRUE] -> w352
      tunnel: w355 -> [w362 w367 w375 w383 w394 w404]
      tunnel: w354 -> [w361 w366 w374 w382 w393 w402]
      tunnel: [w361 w366 w374 w382 w393 w397] -> w353
      tunnel: [w362 w367 w375 w383 w394 w401] -> w349
      event Timeout {
        # "Timeout will execute every 25 ms"
        n100 = event-data() -> ()  [unwired: 1 in, 3 out]
      }
      event "Toggle LED": Mouse Down {
        # "Que T Command"
        # "Toggle button has been activated Que T command"
        n101 = event-data() -> ()  [unwired: 1 in, 8 out]
        n102 = Enqueue Element(queue=w373, element="T", error in (no error)=w371) -> (queue out=w370:refnum<queue>, error out=w369:errorcluster)  [unwired: 1 in, 1 out]
      }
      event "Difficulty.Command A": Mouse Down {
        # "Que A Command"
        # "A Command button has been activated Que A command"
        n103 = event-data() -> ()  [unwired: 1 in, 8 out]
        n104 = Enqueue Element(queue=w381, element="A", error in (no error)=w379) -> (queue out=w378:refnum<queue>, error out=w377:errorcluster)  [unwired: 1 in, 1 out]
      }
      event "Difficulty.Command B": Mouse Down {
        # "Que B Command"
        # "B Command button has been activated Que B command"
        n105 = event-data() -> ()  [unwired: 1 in, 8 out]
        n106 = Enqueue Element(queue=w389, element="B", error in (no error)=w387) -> (queue out=w386:refnum<queue>, error out=w385:errorcluster)  [unwired: 1 in, 1 out]
      }
      event "Difficulty.Command C": Mouse Down {
        # "Que C Command"
        # "C Command button has been activated Que B command"
        n107 = event-data() -> ()  [unwired: 1 in, 8 out]
        n108 = Enqueue Element(queue=w391, element="C", error in (no error)=w390) -> (queue out=w392:refnum<queue>)  [unwired: 1 in, 2 out]
      }
      event "Stop": Value Change {
        # "Stop Application"
        n109 = event-data() -> ()  [unwired: 1 in, 6 out]
        n110 = Enqueue Element(queue=w404, element="S", error in (no error)=w402) -> (queue out=w401:refnum<queue>, error out=w400:errorcluster)  [unwired: 1 in, 1 out]
        n111 = property on="Connected" class="Bool (strict)"(error in=w400, "Value"=FALSE ("Connected")) -> (error out=w398:errorcluster)  [unwired: 1 in, 1 out]
        n112 = property on="Response" class="Str"(error in=w398, "Value"="") -> (error out=w397:errorcluster)  [unwired: 1 in, 1 out]
      }
    }
    n113 = property on="error" class="Bool (strict)"() -> ("Value"=w351:bool)  [unwired: 2 in, 2 out]
    n114 = Or(x=w352, y=w351) -> (x .or. y?=w350:bool)
  }
  n115 = VISA Close(VISA resource name=w14, error in (no error)=w13) -> (error out=w5:errorcluster)
  n116 = property on="error" class="Bool (strict)"() -> ("Value"=w1:bool)  [unwired: 2 in, 2 out]
  n117 = Release Queue(queue=w20, error in (no error)=w18) -> (error out=w4:errorcluster)  [unwired: 1 in, 2 out]
  n118 = Release Queue(queue=w19, error in (no error)=w15) -> (error out=w3:errorcluster)  [unwired: 1 in, 2 out]
  n119 = case shown="False" w1 {
    tunnel: w5 -> [w410 _]
    tunnel: w4 -> [w409 _]
    tunnel: w3 -> [w408 _]
    frame False {
      n120 = call <vilib>:"Simple Error Handler.vi"("error in (no error)"=w410) -> ()  [unwired: 1 in, 8 out]
      n121 = call <vilib>:"Simple Error Handler.vi"("error in (no error)"=w409) -> ()  [unwired: 1 in, 8 out]
      n122 = call <vilib>:"Simple Error Handler.vi"("error in (no error)"=w408) -> ()  [unwired: 1 in, 8 out]
    }
    frame True {
    }
  }
